vi "dfd_Maxflat Build ZPK.vi"(7 "symmetric FIR ? (T)":bool, 8 "error in (no error)":errorcluster, 9 "L":i32=3, 10 "poles":cdb[](array[numeric]), 11 "zeros":cdb[](array[numeric]) format="%#_6e") -> (0 "error out":errorcluster, 1 "poles":cdb[](array[numeric]), 2 "zeros":cdb[](array[numeric]), 5 "gain":dbl)   [LabVIEW 2017, in "NI_DigFilter_Design.lvlib"]
doc: "Builds the filter according to the zeros at z = -1 and the coefficients of polynomial."
uses:
  <vilib>/addons/Digital Filter Design/NI_DigFilter_Design.lvlib
  <vilib>/addons/Digital Filter Design/_Misc.llb/dfd_Error Handlers (Single).vi
  <vilib>/addons/Digital Filter Design/NI_DigFilterLicensed.lvlib
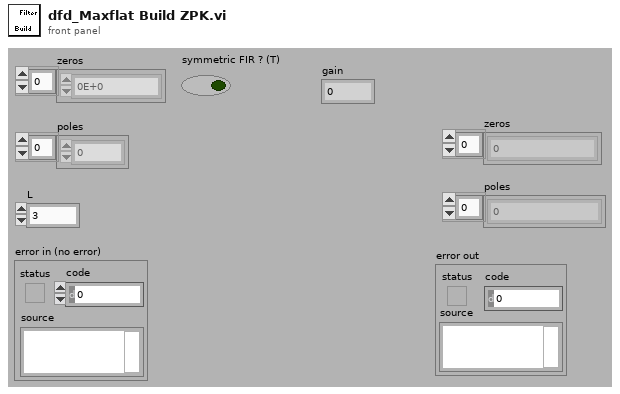
[diagram p1: front panel]
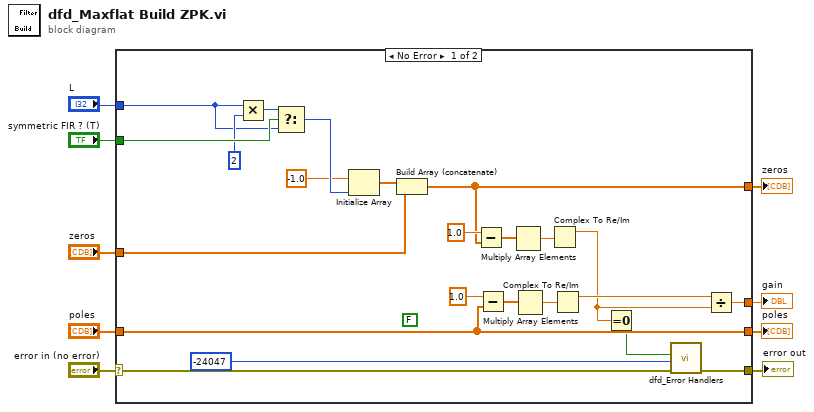
[diagram p0: block diagram]
diagram:
  n1 = case shown="No Error" "error in (no error)" {
    selector: "error in (no error)" -> [w28 w33]
    tunnel: "poles" -> [w19 _]
    tunnel: "zeros" -> [w13 _]
    tunnel: [w14 w33] -> w7
    tunnel: "symmetric FIR ? (T)" -> [w32 _]
    tunnel: "L" -> [w29 _]
    tunnel: [w23 _] -> w2
    tunnel: [w19 _] -> w3
    tunnel: [w15 _] -> w1
    frame No Error {
      (unwired) FALSE ("logical OR")
      n2 = Multiply(x=w29, y=2 ("x")) -> (x*y=w31:i32)
      n3 = Select(t=w31, s=w32, f=w29) -> (s? t:f=w27:i32)
      n4 = Initialize Array(-1.0 ("element"), w27) -> (w25:dbl[])
      n5 = Build Array (concatenate)(w25, w13) -> (w23:cdb[])
      n6 = Subtract(x=1.0, y=w23) -> (x-y=w22:cdb[])
      n7 = Subtract(x=1.0, y=w19) -> (x-y=w21:cdb[])
      n8 = Multiply Array Elements(1:w22) -> (0:w18:cdb)
      n9 = Multiply Array Elements(1:w21) -> (0:w17:cdb)
      n10 = Complex To Re/Im(x + iy=w18) -> (x=w12:dbl)  [unwired: 1 out]
      n11 = Complex To Re/Im(x + iy=w17) -> (x=w16:dbl)  [unwired: 1 out]
      n12 = Equal To 0?(x=w12) -> (x = 0?=w11:bool)
      n13 = call-poly <vilib>:"dfd_Error Handlers.vi"("error in (no error)"=w28, "error code"=-24047 ("ERR_ORDER_BE_LOWER"), "condition failed?"=w11) -> ("error out"=w14:errorcluster)  [unwired: 8 out]
      n14 = Divide(x=w16, y=w12) -> (x/y=w15:dbl)
    }
    frame Error {
    }
  }
  "error out" <- w7
  "zeros" <- w2
  "poles" <- w3
  "gain" <- w1
